vi "Main.vi"(11 "Module Admin":refnum<class "Delacor_lib_QMH_Cloneable Module Admin.lvclass">) -> ()   [LabVIEW 2020, in "Osciloscope Tektronix.lvlib"]
doc: "This template is based off of the Queued Message Handler design pattern and the Queued Message Handler project template that ships with LabVIEW.\n\nThe main difference is that the queue is private to this module and communication between modules is performed via Broadcast and Request events.\n\nRequest events are wrapped in public API methods and are handled in the Event Handling Loop (EHL) of this VI. Any module can register for Broadcast events sent by this module. The EHL generates messages based on user interface actions.\n\nThe Message Handling Loop (MHL) processes messages generated by the EHL, or by other messages. The messages are string values, so new messages can be added easily to the Message Cases case structure in the MHL. Each message cluster can also provide an optional value for Message Data, which is a variant that can be converted to whatever message-specific data is required.\n_____\nBased on DQMH Project Template 6.0.0.91."
uses:
  Osciloscope Tektronix.lvlib
  <vilib>/Delacor/Delacor QMH/Libraries/Cloneable Module Admin_class/Delacor_lib_QMH_Cloneable Module Admin.lvclass
  C:/Program Files (x86)/National Instruments/LabVIEW 2020/vi.lib/Delacor/Delacor QMH/Libraries/Module Admin_class/Delacor_lib_QMH_Module Admin.lvclass
  Module Data--cluster.ctl
  Clases/Implementaciones/Osciloscope/Osciloscope.lvclass
  <vilib>/Delacor/Delacor QMH/Libraries/Message Queue_class/Delacor_lib_QMH_Message Queue.lvclass/Delacor_lib_QMH_Message Queue.ctl
  <vilib>/Delacor/Delacor QMH/Libraries/Cloneable Module Admin_class/Delacor_lib_QMH_Cloneable Module Admin.lvclass/Delacor_lib_QMH_Cloneable Module Admin.ctl
  Stop Argument--cluster.ctl
  <vilib>/Delacor/Delacor QMH/Libraries/Module Admin_class/Delacor_lib_QMH_Module Admin.lvclass/Delacor_lib_QMH_Module Admin.ctl
  SET COM Port Argument--cluster.ctl
  Initialize Oscilloscope Argument--cluster.ctl
  Close Oscilloscope Argument--cluster.ctl
  AutoSetup Argument--cluster.ctl
  Configure Channel Argument--cluster.ctl
  Reset Argument--cluster.ctl
  Read Waveform Argument--cluster.ctl
  Read Waveform (Reply Payload)--cluster.ctl
  Read Measurement Argument--cluster.ctl
  Read Measurement (Reply Payload)--cluster.ctl
  Read Measurement 2 Channels Argument--cluster.ctl
  Read Measurement 2 channels (Reply Payload)--cluster.ctl
  Set Oscilloscope Type Argument--cluster.ctl
  <vilib>/Utility/miscctls.llb/LVPointTypeDef.ctl
  Clases/Implementaciones/Osciloscope/Osciloscope.lvclass/Osciloscope.ctl
  <vilib>/Delacor/Delacor QMH/Libraries/Message Queue_class/Delacor_lib_QMH_Enqueue Message (Single).vi
  <vilib>/Delacor/Delacor QMH/Libraries/Cloneable Module Admin_class/Delacor_lib_QMH_Get Module ID.vi
  <vilib>/Delacor/Delacor QMH/Libraries/Module Admin_class/Delacor_lib_QMH_Get External Launch.vi
  Clases/Implementaciones/Osciloscope/Read COM.vi
  <vilib>/Utility/error.llb/Error Cluster From Error Code.vi
  <vilib>/ErrorRing/Error Ring.xnode
  <vilib>/Delacor/Delacor QMH/Libraries/Message Queue_class/Delacor_lib_QMH_Message Queue.lvclass
panel:
  out "error out":errorcluster
  out "Status":string
  in  "Simulate EHL Error":bool
  in  "Simulate MHL Error":bool
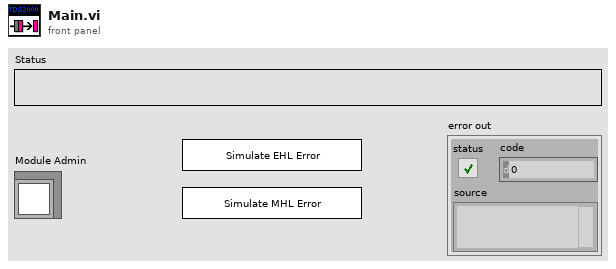
[diagram p1: front panel]
types:
  T1 = typedef "Osciloscope Tektronix.lvlib/Request Events--cluster.ctl" = cluster{"Stop Module":refnum<user-event>, "Show Panel":refnum<user-event>, "Hide Panel":refnum<user-event>, "Show Diagram":refnum<user-event>, "Get Module Execution Status":refnum<user-event>, "SET COM Port":refnum<user-event>, "Initialize Oscilloscope":refnum<user-event>, "Close Oscilloscope":refnum<user-event>, "AutoSetup":refnum<user-event>, "Configure Channel":refnum<user-event>, "Reset":refnum<user-event>, "Read Waveform":refnum<user-event>, "Read Measurement":refnum<user-event>, "Read Measurement 2 channels":refnum<user-event>, "Set Oscilloscope Type":refnum<user-event>}
  T2 = typedef "Osciloscope Tektronix.lvlib/Module Data--cluster.ctl" = cluster{"Status":string, "Osciloscope":refnum<class "Osciloscope.lvclass">}
  T3 = enum32{"invalid lock state", "Not Locked", "Locked (No Password)", "Password-protected"}
  T4 = typedef "Osciloscope Tektronix.lvlib/Stop Argument--cluster.ctl" = cluster{"Module ID":i32, "Origin":string, "Exit via Stop Module Req?":bool, "Wait for Module to stop?":bool}
  T5 = typedef "Osciloscope Tektronix.lvlib/SET COM Port Argument--cluster.ctl" = cluster{"Module ID":i32, "COM":refnum<visa-resource-name>}
  T6 = typedef "Osciloscope Tektronix.lvlib/Initialize Oscilloscope Argument--cluster.ctl" = cluster{"Module ID":i32, "ID Query? (T: Yes)":bool, "Reset? (T: Yes)":bool, "Serial Configuration":cluster{"Baud Rate":u32, "Parity":u16, "Stop Bits":u16, "Flow Control":u16}}
  T7 = typedef "Osciloscope Tektronix.lvlib/Close Oscilloscope Argument--cluster.ctl" = cluster{"Module ID":i32, "Boolean":bool}
  T8 = typedef "Osciloscope Tektronix.lvlib/AutoSetup Argument--cluster.ctl" = cluster{"Module ID":i32, "Boolean":bool}
  T9 = typedef "Osciloscope Tektronix.lvlib/Configure Channel Argument--cluster.ctl" = cluster{"Module ID":i32, "Boolean":bool, "Parameters":cluster{"Enable Channel (True)":bool, "Channel (0: Channel 1)":i32, "Vertical Coupling (1: DC)":i32, "Probe Attenuation (10: 10X)":i32, "Vertical Range (10.0 V/div)":dbl, "Vertical Offset (0.0 divs)":dbl, "Bandwidth (0: MAX Bandwidth)":i32}}
  T10 = typedef "Osciloscope Tektronix.lvlib/Reset Argument--cluster.ctl" = cluster{"Module ID":i32, "Boolean":bool}
  T11 = typedef "Osciloscope Tektronix.lvlib/Read Waveform Argument--cluster.ctl" = cluster{"Module ID":i32, "Wait Notifier":refnum<notifier>, "wait for reply":bool, "Parameters 3":cluster{"Source (0: Channel 1)":u16, "Timeout (10000 ms)":u32}}
  T12 = typedef "Osciloscope Tektronix.lvlib/Read Measurement Argument--cluster.ctl" = cluster{"Module ID":i32, "Wait Notifier":refnum<notifier>, "wait for reply":bool, "Read Parameters":cluster{"Channel (1: Channel 1)":i32, "Measurement Type (0: Frequency)":i32}}
  T13 = typedef "Osciloscope Tektronix.lvlib/Read Measurement 2 channels Argument--cluster.ctl" = cluster{"Module ID":i32, "Wait Notifier":refnum<notifier>, "wait for reply":bool, "Parameters":cluster{"Channel 1 (1: Channel 1)":i32, "Channel 2 (2: Channel 2)":i32, "Measurement Type (0: Phase)":i32}}
  T14 = typedef "Osciloscope Tektronix.lvlib/Set Oscilloscope Type Argument--cluster.ctl" = cluster{"Module ID":i32, "Oscilloscope ":string}
  T15 = typedef "LVPointTypeDef.ctl" = cluster{"Horizontal":i16, "Vertical":i16}
  T16 = enum32{"Invalid", "Standard", "Closed", "Hidden", "Minimized", "Maximized"}
  T17 = typedef "Osciloscope Tektronix.lvlib/Read Waveform (Reply Payload)--cluster.ctl" = cluster{"Read Waveform_error":errorcluster, "Waveform Data":waveform(dbl)}
  T18 = typedef "Osciloscope Tektronix.lvlib/Read Measurement (Reply Payload)--cluster.ctl" = cluster{"Read Measurement_error":errorcluster, "Measurement":dbl, "Units":string}
  T19 = typedef "Osciloscope Tektronix.lvlib/Read Measurement 2 channels (Reply Payload)--cluster.ctl" = cluster{"Read Measurement 2 channels_error":errorcluster, "Measurement":dbl, "Units":string}
  T20 = cluster{"Baud Rate":u32, "Parity":u16, "Stop Bits":u16, "Flow Control":u16}
  T21 = cluster{"Enable Channel (True)":bool, "Channel (0: Channel 1)":i32, "Vertical Coupling (1: DC)":i32, "Probe Attenuation (10: 10X)":i32, "Vertical Range (10.0 V/div)":dbl, "Vertical Offset (0.0 divs)":dbl, "Bandwidth (0: MAX Bandwidth)":i32}
  T22 = cluster{"Source (0: Channel 1)":u16, "Timeout (10000 ms)":u32}
  T23 = cluster{"Channel (1: Channel 1)":i32, "Measurement Type (0: Frequency)":i32}
  T24 = cluster{"Channel 1 (1: Channel 1)":i32, "Channel 2 (2: Channel 2)":i32, "Measurement Type (0: Phase)":i32}
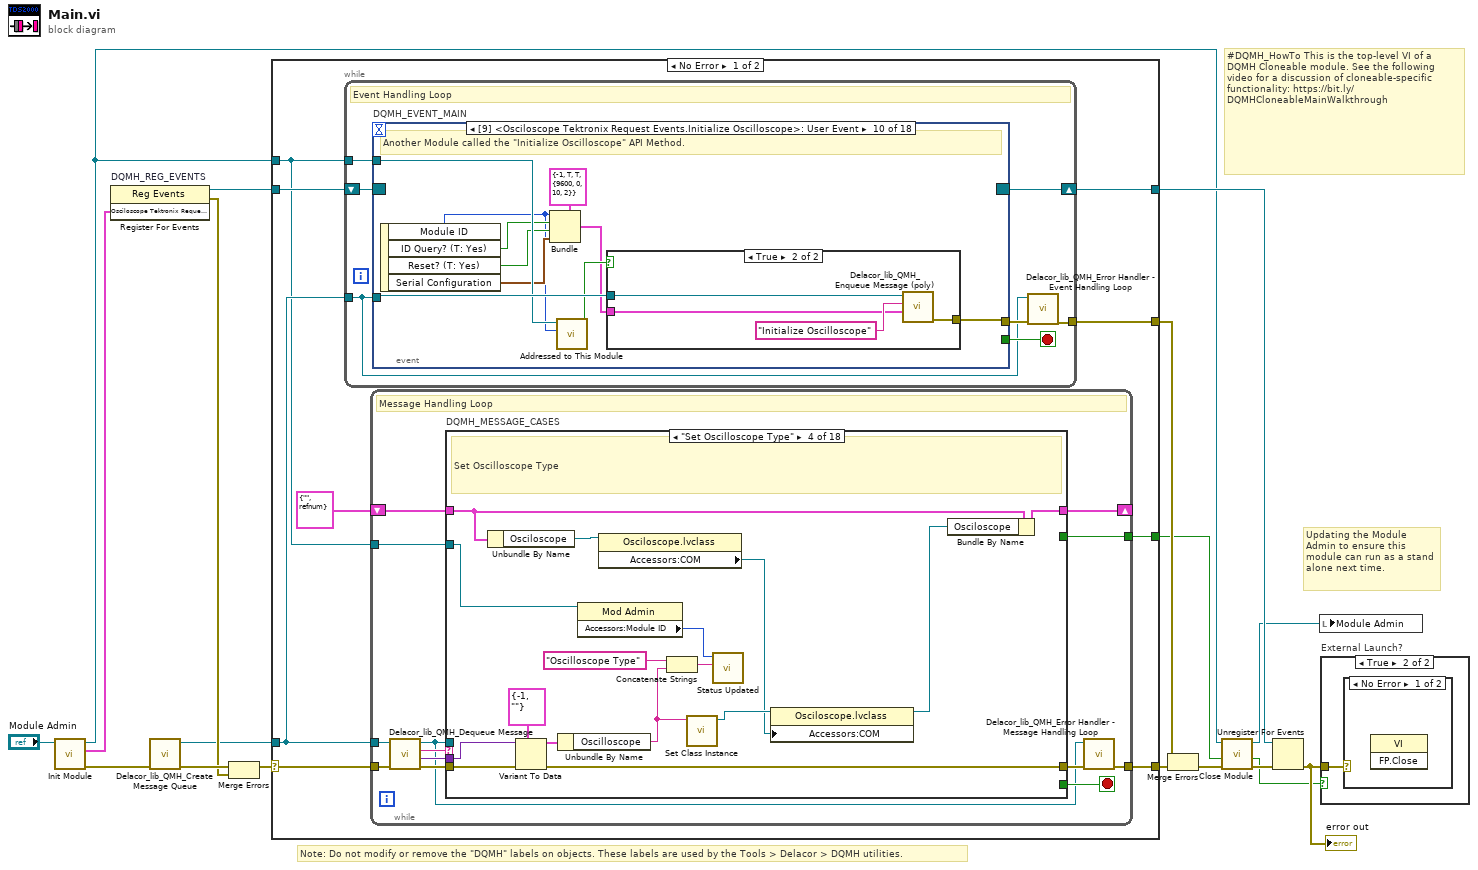
[diagram p0: block diagram]
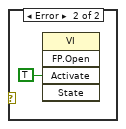
[diagram p3: hidden frame]
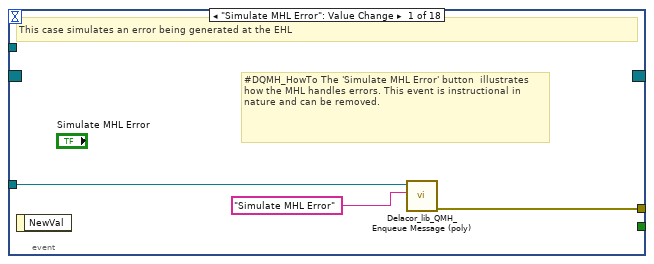
[diagram p4: hidden frame]
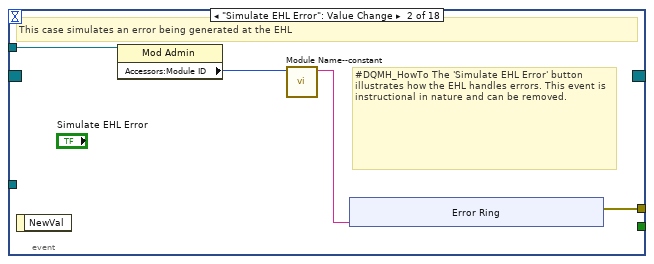
[diagram p5: hidden frame]
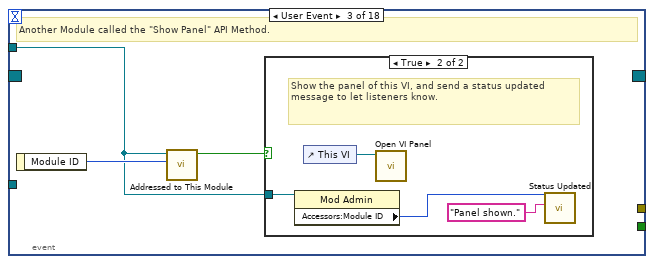
[diagram p6: hidden frame]
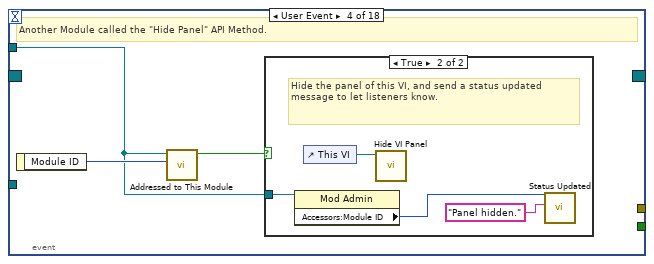
[diagram p8: hidden frame]
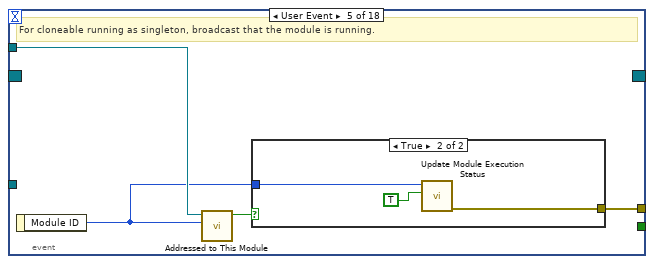
[diagram p10: hidden frame]
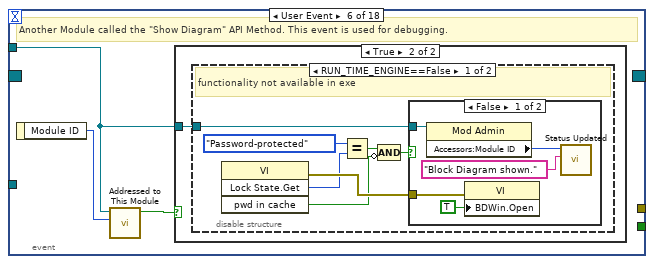
[diagram p12: hidden frame]
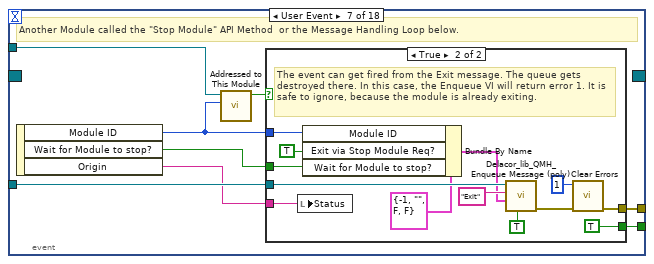
[diagram p16: hidden frame]
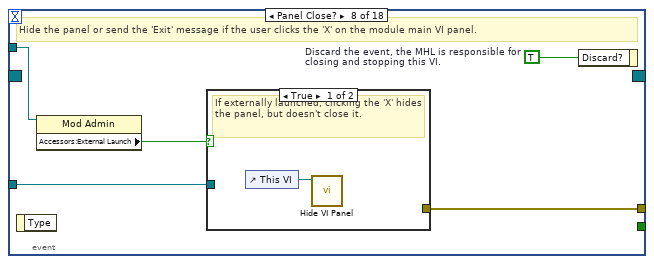
[diagram p18: hidden frame]
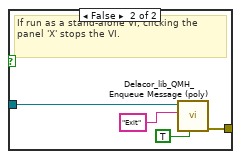
[diagram p19: hidden frame]
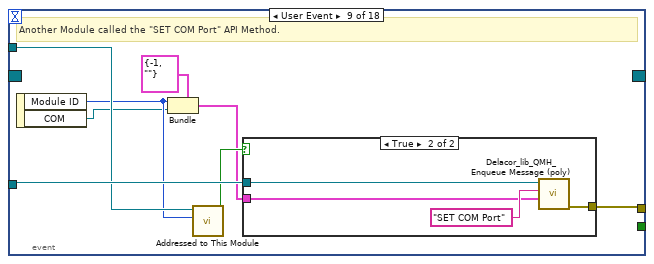
[diagram p20: hidden frame]
diagram:
  # "#DQMH_HowTo This is the top-level VI of a DQMH Cloneable module. See the following video for a discussion of cloneable-specific functionality: https://bit.ly/DQMHCloneableMainWalkthrough"
  # "Note: Do not modify or remove the \"DQMH\" labels on objects. These labels are used by the Tools > Delacor > DQMH utilities."
  # "Updating the Module Admin to ensure this module can run as a stand alone next time."
  n1 = call "Init Module.vi"("Cloneable Module Admin in"="Module Admin") -> ("error out"=w15:errorcluster, "Osciloscope Tektronix Request Events"=w7:T1, "Cloneable Module Admin out"=w4:refnum<class "Delacor_lib_QMH_Cloneable Module Admin.lvclass">)  [unwired: 8 in]
  n2 = register-events "DQMH_REG_EVENTS"(w7) -> (reference out=w8:refnum<event-registration>, error out=w10:errorcluster)  [unwired: 2 in]
  n3 = call <vilib>:"Delacor_lib_QMH_Create Message Queue.vi"("error in"=w15) -> ("error out"=w12:errorcluster, "Message Queue"=w6:refnum<class "Delacor_lib_QMH_Message Queue.lvclass">)  [unwired: 9 in]
  n4 = Merge Errors(w12, w10) -> (w11:errorcluster)
  n5 = case shown="No Error" w11 {
    selector: w11 -> [w25 w512]
    tunnel: [w27 w511] -> w16
    tunnel: [w24 w519] -> w9
    tunnel: w8 -> [w22 w519]
    tunnel: w6 -> [w21 w510]
    tunnel: [w26 _] -> w17
    tunnel: w4 -> [w20 w515]
    tunnel: [w19 _] -> w2
    frame No Error {
      n6 = while {
        tunnel: w21 -> [w28]
        shift-right: [w31] -> w24
        shift-left: w22 -> [w32]
        tunnel: [w33] -> w26
        tunnel: w20 -> [w29]
        stop <- w30 stop-if-true
        # "Event Handling Loop"
        n7 = event "DQMH_EVENT_MAIN" shown="[9] <Osciloscope Tektronix Request Events.Initialize Oscilloscope>: User Event" {
          selector: w32 -> [_ _ _ _ _ _ _ _ _ _ _ _ _ _ _ _ _ _]
          dyn-events: [_ _ _ _ _ _ _ _ _ _ _ _ _ _ _ _ _ _] -> w31
          timeout: _ -> [_ _ _ _ _ _ _ _ _ _ _ _ _ _ _ _ _ _]
          tunnel: [_ _ _ _ _ _ w89 _ _ _ _ _ _ _ _ _ _ _] -> w30
          tunnel: w28 -> [w36 _ _ _ _ _ w92 w108 w124 w138 w150 w162 w175 w187 w201 w215 w229 w241]
          tunnel: [w37 w41 _ _ w66 _ w93 w111 w117 w133 w143 w155 w168 w180 w193 w207 w221 w234] -> w34
          tunnel: w29 -> [_ w40 w49 w56 w64 w70 w91 w109 w122 w136 w148 w160 w173 w185 w199 w213 w227 w239]
          event "Simulate MHL Error": Value Change {
            # "#DQMH_HowTo The 'Simulate MHL Error' button  illustrates how the MHL handles errors. This event is instructional in nature and can be removed."
            # "This case simulates an error being generated at the EHL"
            n8 = event-data() -> ()  [unwired: 1 in, 1 out]
            n9 = call-poly <vilib>:"Delacor_lib_QMH_Enqueue Message (poly).vi"("Message"="Simulate MHL Error", "Message Queue in"=w36) -> ("error out"=w37:errorcluster)  [unwired: 8 in, 1 out]
          }
          event "Simulate EHL Error": Value Change {
            # "#DQMH_HowTo The 'Simulate EHL Error' button  illustrates how the EHL handles errors. This event is instructional in nature and can be removed."
            # "This case simulates an error being generated at the EHL"
            n10 = event-data() -> ()  [unwired: 1 in, 1 out]
            n11 = property class="Mod Admin"(reference=w40) -> ("Accessors:Module ID"=w39:i32)  [unwired: 1 in, 2 out]
            n12 = call "Module Name--constant.vi"("Module ID"=w39) -> ("Module Name"=w38:string)  [unwired: 10 in]
            n13 = xnode "Error Ring"("parameter 0"=w38) -> ("error out"=w41:errorcluster)
          }
          event User Event {
            # "Another Module called the \"Show Panel\" API Method."
            n14 = event-data() -> ("Module ID"=w50:i32)  [unwired: 1 in]
            n15 = call "Addressed to This Module.vi"("Module ID from Argument"=w50, "Module Admin"=w49) -> ("Addressed to this instance?"=w51:bool)  [unwired: 8 in, 1 out]
            n16 = case shown="True" w51 {
              tunnel: w49 -> [_ w53]
              frame False {
              }
              frame True {
                # "Show the panel of this VI, and send a status updated message to let listeners know."
                n17 = property class="Mod Admin"(reference=w53) -> ("Accessors:Module ID"=w52:i32)  [unwired: 1 in, 2 out]
                n18 = control-ref of="This VI"() -> (w55:refnum<vi>)
                n19 = call "Open VI Panel.vi"("VI"=w55) -> ()  [unwired: 10 in, 1 out]
                n20 = call "Status Updated.vi"("Status"="Panel shown." ("format string"), "Module ID"=w52) -> ()  [unwired: 9 in, 1 out]
              }
            }
          }
          event User Event {
            # "Another Module called the \"Hide Panel\" API Method."
            n21 = event-data() -> ("Module ID"=w57:i32)  [unwired: 1 in]
            n22 = call "Addressed to This Module.vi"("Module ID from Argument"=w57, "Module Admin"=w56) -> ("Addressed to this instance?"=w58:bool)  [unwired: 8 in, 1 out]
            n23 = case shown="True" w58 {
              tunnel: w56 -> [_ w60]
              frame False {
              }
              frame True {
                # "Hide the panel of this VI, and send a status updated message to let listeners know."
                n24 = property class="Mod Admin"(reference=w60) -> ("Accessors:Module ID"=w59:i32)  [unwired: 1 in, 2 out]
                n25 = control-ref of="This VI"() -> (w62:refnum<vi>)
                n26 = call "Hide VI Panel.vi"("VI"=w62) -> ()  [unwired: 10 in, 1 out]
                n27 = call "Status Updated.vi"("Status"="Panel hidden." ("format string"), "Module ID"=w59) -> ()  [unwired: 9 in, 1 out]
              }
            }
          }
          event User Event {
            # "For cloneable running as singleton, broadcast that the module is running."
            n28 = event-data() -> ("Module ID"=w63:i32)  [unwired: 1 in]
            n29 = call "Addressed to This Module.vi"("Module ID from Argument"=w63, "Module Admin"=w64) -> ("Addressed to this instance?"=w65:bool)  [unwired: 8 in, 1 out]
            n30 = case shown="True" w65 {
              tunnel: [_ w69] -> w66
              tunnel: w63 -> [_ w68]
              frame False {
              }
              frame True {
                n31 = call "Update Module Execution Status.vi"("Running?"=TRUE, "Module ID"=w68) -> ("error out"=w69:errorcluster)  [unwired: 9 in]
              }
            }
          }
          event User Event {
            # "Another Module called the \"Show Diagram\" API Method. This event is used for debugging."
            n32 = event-data() -> ("Module ID"=w71:i32)  [unwired: 1 in]
            n33 = call "Addressed to This Module.vi"("Module ID from Argument"=w71, "Module Admin"=w70) -> ("Addressed to this instance?"=w72:bool)  [unwired: 8 in, 1 out]
            n34 = case shown="True" w72 {
              tunnel: w70 -> [_ w73]
              frame False {
              }
              frame True {
                n35 = disable-structure shown="RUN_TIME_ENGINE==False" {
                  disable-tunnel: w73 -> [w74 _]
                  frame condition #0 (active) {
                    # "functionality not available in exe"
                    n36 = invoke class="VI" method="Lock State.Get"() -> (error out=w80:errorcluster, "Get Lock State"=w79:T3, "pwd in cache"=w76:bool)  [unwired: 4 in, 1 out]
                    n37 = Equal?(x=T3."Password-protected", y=w79) -> (x = y?=w77:bool)
                    n38 = Compound Arithmetic op=AND(w77, invert w76) -> (w75:bool)
                    n39 = case shown="False" w75 {
                      tunnel: w80 -> [w85 _]
                      tunnel: w74 -> [w82 _]
                      frame False {
                        n40 = property class="Mod Admin"(reference=w82) -> ("Accessors:Module ID"=w81:i32)  [unwired: 1 in, 2 out]
                        n41 = property class="VI"(error in=w85, "BDWin.Open"=TRUE ("Block Diagram Window:Open")) -> ()  [unwired: 1 in, 2 out]
                        n42 = call "Status Updated.vi"("Status"="Block Diagram shown." ("format string"), "Module ID"=w81) -> ()  [unwired: 9 in, 1 out]
                      }
                      frame True {
                        # "Password-protected VI, and the password is not in the cache. Do not show the diagram."
                      }
                    }
                  }
                  frame condition #1 {
                  }
                }
              }
            }
          }
          event User Event {
            # "Another Module called the \"Stop Module\" API Method  or the Message Handling Loop below."
            n43 = event-data() -> ("Module ID"=w87:i32, "Wait for Module to stop?"=w88:bool, "Origin"=w86:string)  [unwired: 1 in]
            n44 = call "Addressed to This Module.vi"("Module ID from Argument"=w87, "Module Admin"=w91) -> ("Addressed to this instance?"=w90:bool)  [unwired: 8 in, 1 out]
            n45 = case shown="True" w90 {
              tunnel: [_ w105] -> w93
              tunnel: w92 -> [_ w101]
              tunnel: [_ TRUE] -> w89
              tunnel: w88 -> [_ w96]
              tunnel: w87 -> [_ w98]
              tunnel: w86 -> [_ w94]
              frame False {
              }
              frame True {
                # "The event can get fired from the Exit message. The queue gets destroyed there. In this case, the Enqueue VI will return error 1. It is safe to ignore, because the module is already exiting."
                n46 = local write "Status"(w94) -> ()
                n47 = Bundle By Name(cluster=T4 {"Module ID"=-1, "Origin"="", "Exit via Stop Module Req?"=FALSE, "Wait for Module to stop?"=FALSE} ("Stop Argument"), "Module ID"=w98, "Exit via Stop Module Req?"=TRUE, "Wait for Module to stop?"=w96) -> (w95:T4)
                n48 = call-poly <vilib>:"Delacor_lib_QMH_Enqueue Message (poly).vi"("Priority Message? (F)"=TRUE, "Message Data"=w95, "Message"="Exit", "Message Queue in"=w101) -> ("error out"=w106:errorcluster)  [unwired: 6 in, 1 out]
                n49 = call <vilib>:"Clear Errors.vi"("error in (no error)"=w106, "specific error code to clear (0: all)"=1) -> ("error out"=w105:errorcluster)  [unwired: 4 in, 1 out]
              }
            }
          }
          event Panel Close? {
            w110 = TRUE  # Discard the event, the MHL is responsible for closing and stopping this VI.
            # "Hide the panel or send the 'Exit' message if the user clicks the 'X' on the module main VI panel."
            n50 = event-data() -> ()  [unwired: 1 in, 1 out]
            n51 = property class="Mod Admin"(reference=w109) -> ("Accessors:External Launch"=w107:bool)  [unwired: 1 in, 2 out]
            n52 = case shown="True" w107 {
              tunnel: w108 -> [_ w115]
              tunnel: [_ w116] -> w111
              frame True {
                # "If externally launched, clicking the 'X' hides the panel, but doesn't close it."
                n53 = control-ref of="This VI"() -> (w112:refnum<vi>)
                n54 = call "Hide VI Panel.vi"("VI"=w112) -> ()  [unwired: 10 in, 1 out]
              }
              frame False {
                # "If run as a stand-alone VI, clicking the panel 'X' stops the VI."
                n55 = call-poly <vilib>:"Delacor_lib_QMH_Enqueue Message (poly).vi"("Priority Message? (F)"=TRUE, "Message"="Exit", "Message Queue in"=w115) -> ("error out"=w116:errorcluster)  [unwired: 7 in, 1 out]
              }
            }
            n56 = event-data("Discard?"=w110) -> ()  [unwired: 1 in, 1 out]
          }
          event User Event {
            # "Another Module called the \"SET COM Port\" API Method."
            n57 = event-data() -> ("Module ID"=w119:i32, "COM"=w118:refnum<visa-resource-name>)  [unwired: 1 in]
            n58 = Bundle(cluster=T5 {"Module ID"=-1, "COM"=""} ("SET COM Port Argument"), "Module ID"=w119, "COM"=w118) -> (w120:T5)
            n59 = call "Addressed to This Module.vi"("Module ID from Argument"=w119, "Module Admin"=w122) -> ("Addressed to this instance?"=w123:bool)  [unwired: 8 in, 1 out]
            n60 = case shown="True" w123 {
              tunnel: w124 -> [_ w128]
              tunnel: w120 -> [_ w126]
              tunnel: [_ w125] -> w117
              frame False {
              }
              frame True {
                n61 = call-poly <vilib>:"Delacor_lib_QMH_Enqueue Message (poly).vi"("Message Data"=w126, "Message"="SET COM Port", "Message Queue in"=w128) -> ("error out"=w125:errorcluster)  [unwired: 7 in, 1 out]
              }
            }
          }
          event User Event {
            # "Another Module called the \"Initialize Oscilloscope\" API Method."
            n62 = event-data() -> ("Module ID"=w129:i32, "ID Query? (T: Yes)"=w131:bool, "Reset? (T: Yes)"=w130:bool, "Serial Configuration"=w132:T20)  [unwired: 1 in]
            n63 = Bundle(cluster=T6 {"Module ID"=-1, "ID Query? (T: Yes)"=TRUE, "Reset? (T: Yes)"=TRUE, "Serial Configuration"={"Baud Rate"=9600, "Parity"=0, "Stop Bits"=10, "Flow Control"=2}} ("Initialize Oscilloscope Argument"), "Module ID"=w129, "ID Query? (T: Yes)"=w131, "Reset? (T: Yes)"=w130, "Serial Configuration"=w132) -> (w134:T6)
            n64 = call "Addressed to This Module.vi"("Module ID from Argument"=w129, "Module Admin"=w136) -> ("Addressed to this instance?"=w137:bool)  [unwired: 8 in, 1 out]
            n65 = case shown="True" w137 {
              tunnel: w138 -> [_ w142]
              tunnel: w134 -> [_ w140]
              tunnel: [_ w139] -> w133
              frame False {
              }
              frame True {
                n66 = call-poly <vilib>:"Delacor_lib_QMH_Enqueue Message (poly).vi"("Message Data"=w140, "Message"="Initialize Oscilloscope", "Message Queue in"=w142) -> ("error out"=w139:errorcluster)  [unwired: 7 in, 1 out]
              }
            }
          }
          event User Event {
            # "Another Module called the \"Close Oscilloscope\" API Method."
            n67 = event-data() -> ("Module ID"=w145:i32, "Boolean"=w144:bool)  [unwired: 1 in]
            n68 = Bundle(cluster=T7 {"Module ID"=-1, "Boolean"=FALSE} ("Close Oscilloscope Argument"), "Module ID"=w145, "Boolean"=w144) -> (w146:T7)
            n69 = call "Addressed to This Module.vi"("Module ID from Argument"=w145, "Module Admin"=w148) -> ("Addressed to this instance?"=w149:bool)  [unwired: 8 in, 1 out]
            n70 = case shown="True" w149 {
              tunnel: w150 -> [_ w154]
              tunnel: w146 -> [_ w152]
              tunnel: [_ w151] -> w143
              frame False {
              }
              frame True {
                n71 = call-poly <vilib>:"Delacor_lib_QMH_Enqueue Message (poly).vi"("Message Data"=w152, "Message"="Close Oscilloscope", "Message Queue in"=w154) -> ("error out"=w151:errorcluster)  [unwired: 7 in, 1 out]
              }
            }
          }
          event User Event {
            # "Another Module called the \"AutoSetup\" API Method."
            n72 = event-data() -> ("Module ID"=w157:i32, "Boolean"=w156:bool)  [unwired: 1 in]
            n73 = Bundle(cluster=T8 {"Module ID"=-1, "Boolean"=FALSE} ("AutoSetup Argument"), "Module ID"=w157, "Boolean"=w156) -> (w158:T8)
            n74 = call "Addressed to This Module.vi"("Module ID from Argument"=w157, "Module Admin"=w160) -> ("Addressed to this instance?"=w161:bool)  [unwired: 8 in, 1 out]
            n75 = case shown="True" w161 {
              tunnel: w162 -> [_ w166]
              tunnel: w158 -> [_ w164]
              tunnel: [_ w163] -> w155
              frame False {
              }
              frame True {
                n76 = call-poly <vilib>:"Delacor_lib_QMH_Enqueue Message (poly).vi"("Message Data"=w164, "Message"="AutoSetup", "Message Queue in"=w166) -> ("error out"=w163:errorcluster)  [unwired: 7 in, 1 out]
              }
            }
          }
          event User Event {
            # "Another Module called the \"Configure Channel\" API Method."
            n77 = event-data() -> ("Module ID"=w170:i32, "Boolean"=w169:bool, "Parameters"=w167:T21)  [unwired: 1 in]
            n78 = Bundle(cluster=T9 {"Module ID"=-1, "Boolean"=FALSE, "Parameters"={"Enable Channel (True)"=TRUE, "Channel (0: Channel 1)"=0, "Vertical Coupling (1: DC)"=1, "Probe Attenuation (10: 10X)"=10, "Vertical Range (10.0 V/div)"=10.0, "Vertical Offset (0.0 divs)"=0.0, "Bandwidth (0: MAX Bandwidth)"=0}} ("Configure Channel Argument"), "Module ID"=w170, "Boolean"=w169, "Parameters"=w167) -> (w171:T9)
            n79 = call "Addressed to This Module.vi"("Module ID from Argument"=w170, "Module Admin"=w173) -> ("Addressed to this instance?"=w174:bool)  [unwired: 8 in, 1 out]
            n80 = case shown="True" w174 {
              tunnel: w175 -> [_ w179]
              tunnel: w171 -> [_ w177]
              tunnel: [_ w176] -> w168
              frame False {
              }
              frame True {
                n81 = call-poly <vilib>:"Delacor_lib_QMH_Enqueue Message (poly).vi"("Message Data"=w177, "Message"="Configure Channel", "Message Queue in"=w179) -> ("error out"=w176:errorcluster)  [unwired: 7 in, 1 out]
              }
            }
          }
          event User Event {
            # "Another Module called the \"Reset\" API Method."
            n82 = event-data() -> ("Module ID"=w182:i32, "Boolean"=w181:bool)  [unwired: 1 in]
            n83 = Bundle(cluster=T10 {"Module ID"=-1, "Boolean"=FALSE} ("Reset Argument"), "Module ID"=w182, "Boolean"=w181) -> (w183:T10)
            n84 = call "Addressed to This Module.vi"("Module ID from Argument"=w182, "Module Admin"=w185) -> ("Addressed to this instance?"=w186:bool)  [unwired: 8 in, 1 out]
            n85 = case shown="True" w186 {
              tunnel: w187 -> [_ w191]
              tunnel: w183 -> [_ w189]
              tunnel: [_ w188] -> w180
              frame False {
              }
              frame True {
                n86 = call-poly <vilib>:"Delacor_lib_QMH_Enqueue Message (poly).vi"("Message Data"=w189, "Message"="Reset", "Message Queue in"=w191) -> ("error out"=w188:errorcluster)  [unwired: 7 in, 1 out]
              }
            }
          }
          event User Event {
            # "Another Module called the \"Read Waveform\" API Method."
            n87 = event-data() -> ("Module ID"=w196:i32, "Wait Notifier"=w195:refnum<notifier>, "wait for reply"=w194:bool, "Parameters 3"=w192:T22)  [unwired: 1 in]
            n88 = Bundle(cluster=T11 {"Module ID"=-1, "Wait Notifier"=refnum, "wait for reply"=FALSE, "Parameters 3"={"Source (0: Channel 1)"=0, "Timeout (10000 ms)"=10000}} ("Read Waveform Argument"), "Module ID"=w196, "Wait Notifier"=w195, "wait for reply"=w194, "Parameters 3"=w192) -> (w197:T11)
            n89 = call "Addressed to This Module.vi"("Module ID from Argument"=w196, "Module Admin"=w199) -> ("Addressed to this instance?"=w200:bool)  [unwired: 8 in, 1 out]
            n90 = case shown="True" w200 {
              tunnel: w201 -> [_ w205]
              tunnel: w197 -> [_ w203]
              tunnel: [_ w202] -> w193
              frame False {
              }
              frame True {
                n91 = call-poly <vilib>:"Delacor_lib_QMH_Enqueue Message (poly).vi"("Message Data"=w203, "Message"="Read Waveform", "Message Queue in"=w205) -> ("error out"=w202:errorcluster)  [unwired: 7 in, 1 out]
              }
            }
          }
          event User Event {
            # "Another Module called the \"Read Measurement\" API Method."
            n92 = event-data() -> ("Module ID"=w210:i32, "Wait Notifier"=w209:refnum<notifier>, "wait for reply"=w208:bool, "Read Parameters"=w206:T23)  [unwired: 1 in]
            n93 = Bundle(cluster=T12 {"Module ID"=-1, "Wait Notifier"=refnum, "wait for reply"=FALSE, "Read Parameters"={"Channel (1: Channel 1)"=1, "Measurement Type (0: Frequency)"=0}} ("Read Measurement Argument"), "Module ID"=w210, "Wait Notifier"=w209, "wait for reply"=w208, "Read Parameters"=w206) -> (w211:T12)
            n94 = call "Addressed to This Module.vi"("Module ID from Argument"=w210, "Module Admin"=w213) -> ("Addressed to this instance?"=w214:bool)  [unwired: 8 in, 1 out]
            n95 = case shown="True" w214 {
              tunnel: w215 -> [_ w219]
              tunnel: w211 -> [_ w217]
              tunnel: [_ w216] -> w207
              frame False {
              }
              frame True {
                n96 = call-poly <vilib>:"Delacor_lib_QMH_Enqueue Message (poly).vi"("Message Data"=w217, "Message"="Read Measurement", "Message Queue in"=w219) -> ("error out"=w216:errorcluster)  [unwired: 7 in, 1 out]
              }
            }
          }
          event User Event {
            # "Another Module called the \"Read Measurement 2 channels\" API Method."
            n97 = event-data() -> ("Module ID"=w224:i32, "Wait Notifier"=w223:refnum<notifier>, "wait for reply"=w222:bool, "Parameters"=w220:T24)  [unwired: 1 in]
            n98 = Bundle(cluster=T13 {"Module ID"=-1, "Wait Notifier"=refnum, "wait for reply"=FALSE, "Parameters"={"Channel 1 (1: Channel 1)"=1, "Channel 2 (2: Channel 2)"=2, "Measurement Type (0: Phase)"=0}} ("Read Measurement 2 channels Argument"), "Module ID"=w224, "Wait Notifier"=w223, "wait for reply"=w222, "Parameters"=w220) -> (w225:T13)
            n99 = call "Addressed to This Module.vi"("Module ID from Argument"=w224, "Module Admin"=w227) -> ("Addressed to this instance?"=w228:bool)  [unwired: 8 in, 1 out]
            n100 = case shown="True" w228 {
              tunnel: w229 -> [_ w233]
              tunnel: w225 -> [_ w231]
              tunnel: [_ w230] -> w221
              frame False {
              }
              frame True {
                n101 = call-poly <vilib>:"Delacor_lib_QMH_Enqueue Message (poly).vi"("Message Data"=w231, "Message"="Read Measurement 2 channels", "Message Queue in"=w233) -> ("error out"=w230:errorcluster)  [unwired: 7 in, 1 out]
              }
            }
          }
          event User Event {
            # "Another Module called the \"Set Oscilloscope Type\" API Method."
            n102 = event-data() -> ("Module ID"=w236:i32, "Oscilloscope"=w235:string)  [unwired: 1 in]
            n103 = Bundle(cluster=T14 {"Module ID"=-1, "Oscilloscope "=""} ("Set Oscilloscope Type Argument"), "Module ID"=w236, "Oscilloscope"=w235) -> (w237:T14)
            n104 = call "Addressed to This Module.vi"("Module ID from Argument"=w236, "Module Admin"=w239) -> ("Addressed to this instance?"=w240:bool)  [unwired: 8 in, 1 out]
            n105 = case shown="True" w240 {
              tunnel: w241 -> [_ w245]
              tunnel: w237 -> [_ w243]
              tunnel: [_ w242] -> w234
              frame False {
              }
              frame True {
                n106 = call-poly <vilib>:"Delacor_lib_QMH_Enqueue Message (poly).vi"("Message Data"=w243, "Message"="Set Oscilloscope Type", "Message Queue in"=w245) -> ("error out"=w242:errorcluster)  [unwired: 7 in, 1 out]
              }
            }
          }
        }
        n107 = call-dynamic "Delacor_lib_QMH_Error Handler - Event Handling Loop.vi"("error in"=w34, "Message Queue in"=w28) -> ("dup error in"=w33:errorcluster)  [unwired: 8 in, 1 out]
      }
      n108 = while {
        tunnel: w21 -> [w249]
        shift-right: [w253] -> _
        shift-left: T2 {"Status"="", "Osciloscope"=refnum} ("Data Cluster") -> [w254]
        tunnel: w25 -> [w257]
        tunnel: [w255] -> w27
        tunnel: w20 -> [w247]
        tunnel: [w246] -> w19
        stop <- w252 stop-if-true
        # "Message Handling Loop"
        n109 = call-dynamic "Delacor_lib_QMH_Dequeue Message.vi"("error in"=w257, "Message Queue in"=w249) -> ("error out"=w256:errorcluster, "Message Data"=w250:variant, "Message"=w251:string, "Message Queue out"=w248:refnum<class "Delacor_lib_QMH_Message Queue.lvclass">)  [unwired: 6 in]
        n110 = case "DQMH_MESSAGE_CASES" shown="\"Set Oscilloscope Type\"" w251 {
          selector: w251 -> [_ _ _ _ _ _ _ _ _ _ _ _ _ _ _ _ _ w497]
          tunnel: w248 -> [_ _ _ _ _ _ _ _ _ _ _ _ _ _ w448 _ w487 _]
          tunnel: w256 -> [w278 w282 w298 w314 w331 w345 w359 w371 w382 w399 w419 w439 w444 w446 w457 w470 w493 w499]
          tunnel: [w276 w282 w293 w313 w324 w338 w350 w365 w377 w390 w410 w430 w443 w446 w453 w469 w490 w500] -> w258
          tunnel: w254 -> [w269 w281 w290 w308 w321 w336 w354 w364 w375 w388 w408 w429 w442 w445 w452 w467 w486 w498]
          tunnel: [w268 w281 w289 w309 w326 w335 w353 w363 w374 w387 w407 w428 w442 w445 w452 w467 w486 w498] -> w253
          tunnel: [_ _ _ _ _ _ _ _ _ _ _ _ _ _ _ _ w485 _] -> w252
          tunnel: w250 -> [_ _ w296 w312 w329 w343 w357 w369 w380 w397 w417 w437 _ _ w451 _ w483 _]
          tunnel: w247 -> [w264 _ w286 w304 w315 w334 w346 _ _ _ _ _ _ _ w450 w465 w479 w495]
          tunnel: [_ _ _ _ _ _ _ _ _ _ _ _ _ _ _ _ w481 _] -> w246
          frame "Initialize" {
            w261 = "Initial Message" ("Initial Message")
            # "Initialize - Any operation that needs to be done before the module can receive messages. Synchronize Caller Events.vi will inform Start Module.vi that the module has launched and is ready to receive messages. Module Did Init.vi will broadcast that the module initialized."
            n111 = call "Synchronize Caller Events.vi"("error in (no error)"=w278, "Module Admin"=w264) -> ("error out"=w277:errorcluster, "Module Admin out"=w263:refnum<class "Delacor_lib_QMH_Cloneable Module Admin.lvclass">)  [unwired: 8 in]
            n112 = property class="Mod Admin"(reference=w263) -> ("Accessors:Module ID"=w260:i32, "Accessors:External Launch"=w265:bool)  [unwired: 1 in, 2 out]
            n113 = call "Get Classes Names.vi"() -> ("Classes"=w259:string[])  [unwired: 11 in]
            n114 = call "Oscilloscopes List.vi"("Oscilloscopes Types"=w259, "Module ID"=w260) -> ()  [unwired: 9 in, 1 out]
            n115 = call "Module Name--constant.vi"("Module ID"=w260) -> ("Module Name"=w273:string)  [unwired: 10 in]
            n116 = property class="VI"("Front Panel.Title"=w273) -> (reference out=w275:refnum<vi>, error out=w280:errorcluster)  [unwired: 2 in]
            n117 = Select(t=T16."Hidden" ("State"), s=w265, f=T16."Standard" ("State")) -> (s? t:f=w270:T16)
            n118 = invoke class="VI" method="FP.Open"(reference=w275, error in=w280, "State"=w270) -> (reference out=w274:refnum<vi>, error out=w279:errorcluster)  [unwired: 2 in, 3 out]
            n119 = call "Module Name--constant.vi"("Module ID"=w260) -> ("Module Name"=w266:string)  [unwired: 10 in]
            n120 = Bundle By Name(cluster=w269, "Status"=w261) -> (w268:T2)
            n121 = invoke class="VI" method="FP.Center"(reference=w274, error in=w279) -> ()  [unwired: 1 in, 3 out]
            n122 = property on="Pane" class="Pane"("Origin"=T15 {"Horizontal"=0, "Vertical"=0}) -> ()  [unwired: 2 in, 2 out]
            n123 = call "Module Did Init.vi"("error in (no error)"=w277, "Initialized?"=TRUE, "Origin"=w266, "Module ID"=w260) -> ("error out"=w276:errorcluster)  [unwired: 7 in]
            "Status" <- w261
          }
          frame "---Module Specific---" {
            # "Separator -- The following cases handle messages specific to this Module."
          }
          frame "SET COM Port" {
            # "Set the Visa COM Port"
            n124 = Variant To Data(error in=w298, type=T5 {"Module ID"=-1, "COM"=""} ("SET COM Port Argument"), Variant=w296) -> (data=w294:T5, error out=w297:errorcluster)
            n125 = property class="Mod Admin"(reference=w286) -> ("Accessors:Module ID"=w287:i32)  [unwired: 1 in, 2 out]
            n126 = Unbundle By Name(w294) -> ("COM"=w283:refnum<visa-resource-name>)
            n127 = Unbundle By Name(w290) -> ("Osciloscope"=w291:refnum<class "Osciloscope.lvclass">)
            n128 = Concatenate Strings("COM SET TO:" ("Status"), w283) -> (w284:string)
            n129 = call "Status Updated.vi"("Status"=w284, "Module ID"=w287) -> ()  [unwired: 9 in, 1 out]
            n130 = call "Write COM.vi"("COM"=w283, "Osciloscope in"=w291) -> ("error out"=w292:errorcluster, "Osciloscope out"=w288:refnum<class "Osciloscope.lvclass">)  [unwired: 8 in]
            n131 = Bundle By Name(cluster=w290, "Osciloscope"=w288) -> (w289:T2)
            n132 = Merge Errors(w297, w292) -> (w293:errorcluster)
          }
          frame "Set Oscilloscope Type" {
            # "Set Oscilloscope Type"
            n133 = Unbundle By Name(w308) -> ("Osciloscope"=w307:refnum<class "Osciloscope.lvclass">)
            n134 = Variant To Data(error in=w314, type=T14 {"Module ID"=-1, "Oscilloscope "=""} ("Set Oscilloscope Type Argument"), Variant=w312) -> (data=w310:T14, error out=w313:errorcluster)
            n135 = Unbundle By Name(w310) -> ("Oscilloscope"=w302:string)
            n136 = property class="Mod Admin"(reference=w304) -> ("Accessors:Module ID"=w306:i32)  [unwired: 1 in, 2 out]
            n137 = property class="Osciloscope.lvclass"(reference=w307) -> ("Accessors:COM"=w299:refnum<visa-resource-name>)  [unwired: 1 in, 2 out]
            n138 = Concatenate Strings("Oscilloscope Type" ("Status"), w302) -> (w303:string)
            n139 = call "Set Class Instance.vi"("OsciloscopeType"=w302) -> ("specific class reference"=w301:refnum<class "Osciloscope.lvclass">)  [unwired: 10 in]
            n140 = call "Status Updated.vi"("Status"=w303, "Module ID"=w306) -> ()  [unwired: 9 in, 1 out]
            n141 = property class="Osciloscope.lvclass"(reference=w301, "Accessors:COM"=w299) -> (reference out=w300:refnum<class "Osciloscope.lvclass">)  [unwired: 1 in, 1 out]
            n142 = Bundle By Name(cluster=w308, "Osciloscope"=w300) -> (w309:T2)
          }
          frame "Initialize Oscilloscope" {
            # "Initialize the oscilloscope selected"
            n143 = Variant To Data(error in=w331, type=T6 {"Module ID"=-1, "ID Query? (T: Yes)"=TRUE, "Reset? (T: Yes)"=TRUE, "Serial Configuration"={"Baud Rate"=9600, "Parity"=0, "Stop Bits"=10, "Flow Control"=2}} ("Initialize Oscilloscope Argument"), Variant=w329) -> (data=w327:T6, error out=w330:errorcluster)
            n144 = Unbundle By Name(w321) -> ("Osciloscope"=w318:refnum<class "Osciloscope.lvclass">)
            n145 = Unbundle By Name(w327) -> ("Serial Configuration"=w322:T20, "Reset? (T: Yes)"=w320:bool, "ID Query? (T: Yes)"=w319:bool)
            n146 = property class="Mod Admin"(reference=w315) -> ("Accessors:Module ID"=w317:i32)  [unwired: 1 in, 2 out]
            n147 = call "Status Updated.vi"("Status"="Oscilloscope Init", "Module ID"=w317) -> ()  [unwired: 9 in, 1 out]
            n148 = call-dynamic "Initial.vi"("Serial Configuration"=w322, "ID Query? (T: Yes)"=w319, "Reset? (T: Yes)"=w320, "Osciloscope in"=w318) -> ("error out"=w323:errorcluster, "Osciloscope out"=w325:refnum<class "Osciloscope.lvclass">)  [unwired: 6 in]
            n149 = Bundle By Name(cluster=w321, "Osciloscope"=w325) -> (w326:T2)
            n150 = Merge Errors(w323, w330) -> (w324:errorcluster)
          }
          frame "Close Oscilloscope" {
            # "Close the selected Oscilloscope"
            n151 = Variant To Data(error in=w345, type=T7 {"Module ID"=-1, "Boolean"=FALSE} ("Close Oscilloscope Argument"), Variant=w343) -> (data=w341:T7, error out=w344:errorcluster)
            n152 = property class="Mod Admin"(reference=w334) -> ("Accessors:Module ID"=w333:i32)  [unwired: 1 in, 2 out]
            n153 = Unbundle By Name(w341) -> ()  [unwired: 1 out]
            n154 = Unbundle By Name(w336) -> ("Osciloscope"=w339:refnum<class "Osciloscope.lvclass">)
            n155 = call "Status Updated.vi"("Status"="Oscilloscope Closed", "Module ID"=w333) -> ()  [unwired: 9 in, 1 out]
            n156 = call-dynamic "Close Oscilloscope.vi"("Osciloscope in"=w339) -> ("error out"=w337:errorcluster, "Osciloscope out"=w340:refnum<class "Osciloscope.lvclass">)  [unwired: 9 in]
            n157 = Bundle By Name(cluster=w336, "Osciloscope"=w340) -> (w335:T2)
            n158 = Merge Errors(w344, w337) -> (w338:errorcluster)
          }
          frame "AutoSetup" {
            # "AutoSetup the selected oscilloscope"
            n159 = Variant To Data(error in=w359, type=T8 {"Module ID"=-1, "Boolean"=FALSE} ("AutoSetup Argument"), Variant=w357) -> (data=w355:T8, error out=w358:errorcluster)
            n160 = Unbundle By Name(w354) -> ("Osciloscope"=w352:refnum<class "Osciloscope.lvclass">)
            n161 = property class="Mod Admin"(reference=w346) -> ("Accessors:Module ID"=w348:i32)  [unwired: 1 in, 2 out]
            n162 = Unbundle By Name(w355) -> ()  [unwired: 1 out]
            n163 = call "Status Updated.vi"("Status"="Auto Setup", "Module ID"=w348) -> ()  [unwired: 9 in, 1 out]
            n164 = call-dynamic "Autosetup.vi"("Osciloscope in"=w352) -> ("error out"=w349:errorcluster, "Osciloscope out"=w351:refnum<class "Osciloscope.lvclass">)  [unwired: 9 in]
            n165 = Bundle By Name(cluster=w354, "Osciloscope"=w351) -> (w353:T2)
            n166 = Merge Errors(w358, w349) -> (w350:errorcluster)
          }
          frame "Configure Channel" {
            # "Configure the channels from the selected oscilloscope"
            n167 = Variant To Data(error in=w371, type=T9 {"Module ID"=-1, "Boolean"=FALSE, "Parameters"={"Enable Channel (True)"=TRUE, "Channel (0: Channel 1)"=0, "Vertical Coupling (1: DC)"=1, "Probe Attenuation (10: 10X)"=10, "Vertical Range (10.0 V/div)"=10.0, "Vertical Offset (0.0 divs)"=0.0, "Bandwidth (0: MAX Bandwidth)"=0}} ("Configure Channel Argument"), Variant=w369) -> (data=w367:T9, error out=w370:errorcluster)
            n168 = Unbundle By Name(w367) -> ("Parameters"=w366:T21)
            n169 = Unbundle By Name(w364) -> ("Osciloscope"=w360:refnum<class "Osciloscope.lvclass">)
            n170 = call-dynamic "Configure Channel.vi"("Parameters"=w366, "Osciloscope in"=w360) -> ("error out"=w362:errorcluster, "Osciloscope out"=w361:refnum<class "Osciloscope.lvclass">)  [unwired: 8 in]
            n171 = Bundle By Name(cluster=w364, "Osciloscope"=w361) -> (w363:T2)
            n172 = Merge Errors(w370, w362) -> (w365:errorcluster)
          }
          frame "Reset" {
            # "Reset the selected Oscilloscope"
            n173 = Variant To Data(error in=w382, type=T10 {"Module ID"=-1, "Boolean"=FALSE} ("Reset Argument"), Variant=w380) -> (data=w378:T10, error out=w381:errorcluster)
            n174 = Unbundle By Name(w378) -> ()  [unwired: 1 out]
            n175 = Unbundle By Name(w375) -> ("Osciloscope"=w372:refnum<class "Osciloscope.lvclass">)
            n176 = call-dynamic "Reset.vi"("Osciloscope in"=w372) -> ("error out"=w376:errorcluster, "Osciloscope out"=w373:refnum<class "Osciloscope.lvclass">)  [unwired: 9 in]
            n177 = Bundle By Name(cluster=w375, "Osciloscope"=w373) -> (w374:T2)
            n178 = Merge Errors(w381, w376) -> (w377:errorcluster)
          }
          frame "Read Waveform" {
            n179 = Variant To Data(error in=w399, type=T11 {"Module ID"=-1, "Wait Notifier"=refnum, "wait for reply"=FALSE, "Parameters 3"={"Source (0: Channel 1)"=0, "Timeout (10000 ms)"=10000}} ("Read Waveform Argument"), Variant=w397) -> (data=w395:T11, error out=w398:errorcluster)
            n180 = Unbundle By Name(w388) -> ("Osciloscope"=w389:refnum<class "Osciloscope.lvclass">)
            n181 = Unbundle By Name(w395) -> ("Parameters 3"=w383:T22, "Wait Notifier"=w394:refnum<notifier>, "wait for reply"=w393:bool)
            n182 = call-dynamic "Read Waveform.vi"("Parameters 3"=w383, "Osciloscope in"=w389) -> ("error out"=w385:errorcluster, "Waveform Data"=w384:waveform(dbl), "Osciloscope out"=w386:refnum<class "Osciloscope.lvclass">)  [unwired: 7 in]
            n183 = Merge Errors(w398, w385) -> (w390:errorcluster)
            n184 = Bundle By Name(cluster=T17 {"Read Waveform_error"={"status"=FALSE, "code"=0, "source"=""}, "Waveform Data"={"t0"=timestamp(0 s since 1904-01-01), "dt"=1.0, "Y"=[]}} ("Read Waveform (Reply Payload)"), "Waveform Data"=w384) -> (w392:T17)
            n185 = Bundle By Name(cluster=w388, "Osciloscope"=w386) -> (w387:T2)
            n186 = case shown="True" w393 {
              tunnel: w394 -> [_ w401]
              tunnel: w392 -> [_ w400]
              frame False {
              }
              frame True {
                n187 = Send Notification(notification=w400, notifier=w401) -> ()  [unwired: 1 in, 2 out]
              }
            }
          }
          frame "Read Measurement" {
            n188 = Variant To Data(error in=w419, type=T12 {"Module ID"=-1, "Wait Notifier"=refnum, "wait for reply"=FALSE, "Read Parameters"={"Channel (1: Channel 1)"=1, "Measurement Type (0: Frequency)"=0}} ("Read Measurement Argument"), Variant=w417) -> (data=w415:T12, error out=w418:errorcluster)
            n189 = Unbundle By Name(w408) -> ("Osciloscope"=w406:refnum<class "Osciloscope.lvclass">)
            n190 = Unbundle By Name(w415) -> ("Read Parameters"=w404:T23, "Wait Notifier"=w414:refnum<notifier>, "wait for reply"=w413:bool)
            n191 = call-dynamic "Read Measurement.vi"("Read Parameters"=w404, "Osciloscope in"=w406) -> ("error out"=w409:errorcluster, "Units"=w402:string, "Measurement"=w403:dbl, "Osciloscope out"=w405:refnum<class "Osciloscope.lvclass">)  [unwired: 6 in]
            n192 = Merge Errors(w418, w409) -> (w410:errorcluster)
            n193 = Bundle By Name(cluster=w408, "Osciloscope"=w405) -> (w407:T2)
            n194 = Bundle By Name(cluster=T18 {"Read Measurement_error"={"status"=FALSE, "code"=0, "source"=""}, "Measurement"=0.0, "Units"=""} ("Read Measurement (Reply Payload)"), "Measurement"=w403, "Units"=w402) -> (w412:T18)
            n195 = case shown="True" w413 {
              tunnel: w414 -> [_ w421]
              tunnel: w412 -> [_ w420]
              frame False {
              }
              frame True {
                n196 = Send Notification(notification=w420, notifier=w421) -> ()  [unwired: 1 in, 2 out]
              }
            }
          }
          frame "Read Measurement 2 channels" {
            n197 = Variant To Data(error in=w439, type=T13 {"Module ID"=-1, "Wait Notifier"=refnum, "wait for reply"=FALSE, "Parameters"={"Channel 1 (1: Channel 1)"=1, "Channel 2 (2: Channel 2)"=2, "Measurement Type (0: Phase)"=0}} ("Read Measurement 2 channels Argument"), Variant=w437) -> (data=w435:T13, error out=w438:errorcluster)
            n198 = Unbundle By Name(w435) -> ("Parameters"=w425:T24, "Wait Notifier"=w434:refnum<notifier>, "wait for reply"=w433:bool)
            n199 = Unbundle By Name(w429) -> ("Osciloscope"=w426:refnum<class "Osciloscope.lvclass">)
            n200 = call-dynamic "Read Measurement 2 Channels.vi"("Parameters"=w425, "Osciloscope in"=w426) -> ("error out"=w424:errorcluster, "Units"=w423:string, "Measurement"=w422:dbl, "Osciloscope out"=w427:refnum<class "Osciloscope.lvclass">)  [unwired: 6 in]
            n201 = Merge Errors(w438, w424) -> (w430:errorcluster)
            n202 = Bundle By Name(cluster=T19 {"Read Measurement 2 channels_error"={"status"=FALSE, "code"=0, "source"=""}, "Measurement"=0.0, "Units"=""} ("Read Measurement 2 channels (Reply Payload)"), "Measurement"=w422, "Units"=w423) -> (w432:T19)
            n203 = Bundle By Name(cluster=w429, "Osciloscope"=w427) -> (w428:T2)
            n204 = case shown="True" w433 {
              tunnel: w434 -> [_ w441]
              tunnel: w432 -> [_ w440]
              frame False {
              }
              frame True {
                n205 = Send Notification(notification=w440, notifier=w441) -> ()  [unwired: 1 in, 2 out]
              }
            }
          }
          frame "---Copy This Frame---" {
            # "Duplicate this frame when creating new messages.  Change this comment in the duplicated frame to describe this message."
            n206 = Merge Errors(w444) -> (w443:errorcluster)
          }
          frame "---Exit and Error Handling---" {
            # "Separator - the following cases handle errors and exit messages."
          }
          frame "Error" {
            # "#CodeRecommended - If you ever change the name of this \"Error\" message, you'll need to update the name in the Check Loop Error.vi as well."
            # "#CodeRecommended - If the module is running in standalone mode (External Launch = FALSE), this code will pop up an error dialog and call the 'Exit' message if an error occurs. Add more fine-grained error handling here."
            # "Error - Check the error message data and respond accordingly. This message is sent by the \"Error Handler\" VIs at the end of each loop in this application."
            n207 = property class="Mod Admin"(reference=w450) -> ("Accessors:External Launch"=w449:bool, "Accessors:Module ID"=w447:i32)  [unwired: 1 in, 2 out]
            n208 = Variant To Data(error in=w457, type=errorcluster {"status"=FALSE, "code"=0, "source"=""} ("error constant"), Variant=w451) -> (data=w458:errorcluster, error out=w455:errorcluster)
            n209 = call "Error Reported.vi"("Error"=w458, "Module ID"=w447) -> ()  [unwired: 9 in, 1 out]
            n210 = case shown="False" w449 {
              tunnel: [w463 _] -> w454
              tunnel: w448 -> [w461 _]
              tunnel: w458 -> [w462 _]
              frame False {
                # "If the module is running standalone, then pop up an error dialog and call the \"Exit\" message."
                n211 = call <vilib>:"Simple Error Handler.vi"("error in (no error)"=w462) -> ()  [unwired: 4 in, 5 out]
                n212 = call-poly <vilib>:"Delacor_lib_QMH_Enqueue Message (poly).vi"("Priority Message? (F)"=TRUE, "Message"="Exit", "Message Queue in"=w461) -> ("error out"=w463:errorcluster)  [unwired: 7 in, 1 out]
              }
              frame True {
                # "If the module was launched externally, calling the Error Reported broadcast VI is the only action performed by the \"Error\" message. The module's caller can then process the error appropriately."
              }
            }
            n213 = Merge Errors(w455, w454) -> (w453:errorcluster)
            n214 = local write "error out"(w453) -> ()
          }
          frame "Simulate MHL Error" {
            # "#DQMH_HowTo The 'Simulate MHL Error' button  illustrates how the MHL handles errors. This event is instructional in nature and can be removed."
            # "Simulate an error occurring at the MHL"
            n215 = property class="Mod Admin"(reference=w465) -> ("Accessors:Module ID"=w466:i32)  [unwired: 1 in, 2 out]
            n216 = call "Module Name--constant.vi"("Module ID"=w466) -> ("Module Name"=w464:string)  [unwired: 10 in]
            n217 = xnode "Error Ring"("parameter 0"=w464) -> ("error out"=w468:errorcluster)
            n218 = Merge Errors(w470, w468) -> (w469:errorcluster)
          }
          frame "Exit" {
            w484 = 91  # 91: not all Exit messages will have an argument
            w485 = TRUE  # Stop the VI
            # "Release the message queue reference"
            # "#CodeNeeded - Add any required cleanup code here."
            # "Exit - Exit the application."
            n219 = Variant To Data(error in=w493, type=T4 {"Module ID"=-1, "Origin"="", "Exit via Stop Module Req?"=FALSE, "Wait for Module to stop?"=FALSE} ("Stop Argument"), Variant=w483) -> (data=w480:T4, error out=w488:errorcluster)
            n220 = call <vilib>:"Clear Errors.vi"("error in (no error)"=w488, "specific error code to clear (0: all)"=w484) -> ("error out"=w492:errorcluster)  [unwired: 4 in, 1 out]
            n221 = control-ref of="This VI"() -> (w478:refnum<vi>)
            n222 = call-dynamic "Delacor_lib_QMH_Release Message Queue.vi"("error in"=w492, "Message Queue"=w487) -> ("error out"=w491:errorcluster)  [unwired: 9 in]
            n223 = call "Handle Exit.vi"("Stop Argument"=w480, "Module Admin in"=w479, "VI reference"=w478) -> ("error out"=w489:errorcluster, "Wait for Stop?"=w481:bool)  [unwired: 7 in]
            n224 = Merge Errors(w491, w489) -> (w490:errorcluster)
          }
          frame Default {
            # "'Default' case only runs if there is a message that isn't defined in any of the other cases.  Output a programming error."
            n225 = property class="Mod Admin"(reference=w495) -> ("Accessors:Module ID"=w494:i32)  [unwired: 1 in, 2 out]
            n226 = call "Module Name--constant.vi"("Module ID"=w494) -> ("Module Name"=w496:string)  [unwired: 10 in]
            n227 = xnode "Error Ring"("parameter 0"=w497, "parameter 1"=w496) -> ("error out"=w501:errorcluster)
            n228 = Merge Errors(w499, w501) -> (w500:errorcluster)
          }
        }
        n229 = call-dynamic "Delacor_lib_QMH_Error Handler - Message Handling Loop.vi"("error in"=w258, "Message Queue in"=w248) -> ("dup error in"=w255:errorcluster)  [unwired: 8 in, 1 out]
      }
    }
    frame Error {
      n230 = call "Synchronize Caller Events.vi"("Module Admin"=w515) -> ("Module Admin out"=w514:refnum<class "Delacor_lib_QMH_Cloneable Module Admin.lvclass">)  [unwired: 9 in, 1 out]
      n231 = property class="Mod Admin"(reference=w514) -> ("Accessors:Module ID"=w513:i32)  [unwired: 1 in, 2 out]
      n232 = call-dynamic "Delacor_lib_QMH_Release Message Queue.vi"("error in"=w512, "Message Queue"=w510) -> ("error out"=w511:errorcluster)  [unwired: 9 in]
      n233 = call "Module Name--constant.vi"("Module ID"=w513) -> ("Module Name"=w518:string)  [unwired: 10 in]
      n234 = Format Into String(format string="An error occurred during initialization. %s is no longer running.", w518) -> (resulting string=w516:string)  [unwired: 2 in, 1 out]
      n235 = call "Error Reported.vi"("Additional Information"=w516, "Error"=w511, "Module ID"=w513) -> ()  [unwired: 8 in, 1 out]
    }
  }
  n236 = Merge Errors(w17, w16) -> (w18:errorcluster)
  n237 = call "Close Module.vi"("error in"=w18, "Wait for stop?"=w2, "Module Admin in"=w4) -> ("error out"=w14:errorcluster, "External Launch"=w1:bool, "Module Admin out"=w3:refnum<class "Delacor_lib_QMH_Cloneable Module Admin.lvclass">)  [unwired: 6 in]
  n238 = Unregister For Events(event registration refnum=w9, error in=w14) -> (error out=w13:errorcluster)
  "error out" <- w13
  n239 = local write "Module Admin"(w3) -> ()
  n240 = case "External Launch?" shown="True" w1 {
    tunnel: w13 -> [_ w520]
    frame False {
    }
    frame True {
      n241 = case shown="No Error" w520 {
        frame No Error {
          n242 = invoke class="VI" method="FP.Close"() -> ()  [unwired: 3 in, 3 out]
        }
        frame Error {
          n243 = invoke class="VI" method="FP.Open"("Activate"=TRUE ("Activate?")) -> ()  [unwired: 4 in, 5 out]
        }
      }
    }
  }
